vi "GFITS_Str2EXtensions.vi"(8 "error in":errorcluster, 10 "command":string, 11 "curr_ext":i32) -> (0 "error IO":errorcluster, 1 "max_ext":u16=128, 2 "Extensions":i32[](array[numeric]), 3 "geom extensions":i32[](array[numeric]))   [LabVIEW 2016]
panel:
  out "output array":i32[](array[numeric])
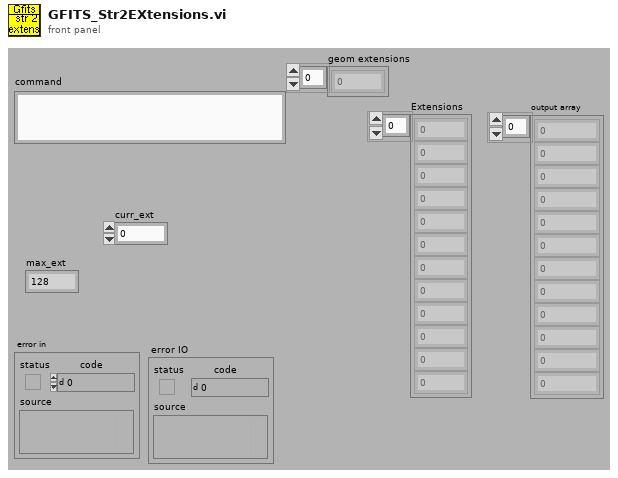
[diagram p1: front panel]
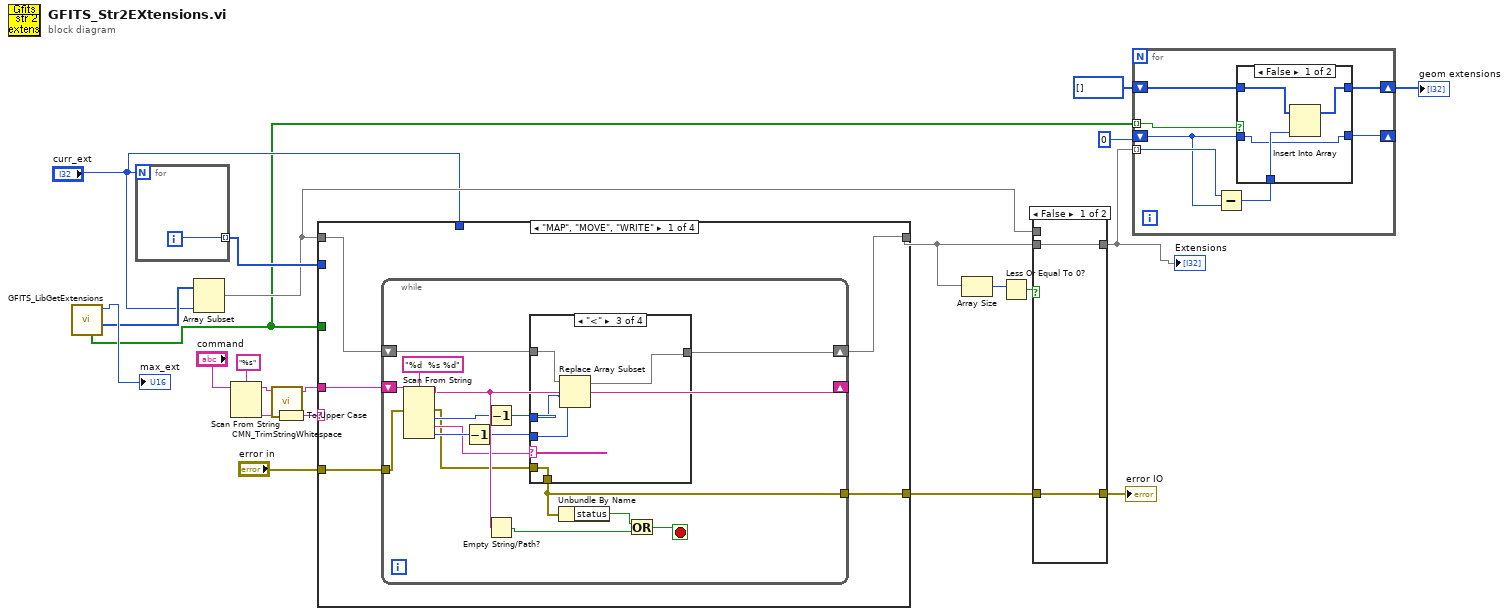
[diagram p0: block diagram]
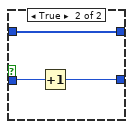
[diagram p2: hidden frame]
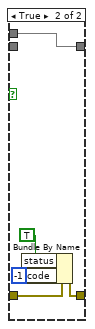
[diagram p3: hidden frame]
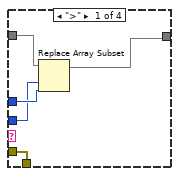
[diagram p4: hidden frame]
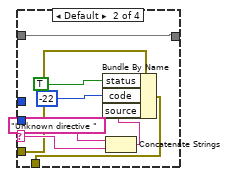
[diagram p5: hidden frame]
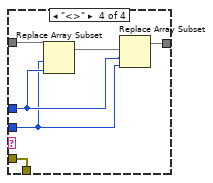
[diagram p6: hidden frame]
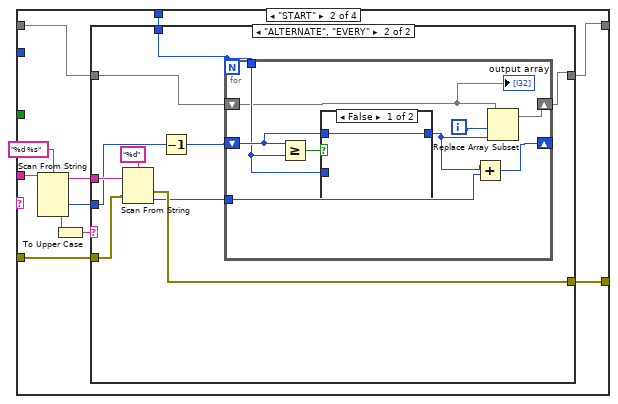
[diagram p7: hidden frame]
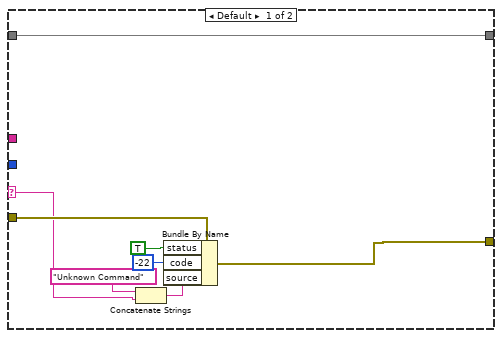
[diagram p8: hidden frame]
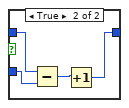
[diagram p9: hidden frame]
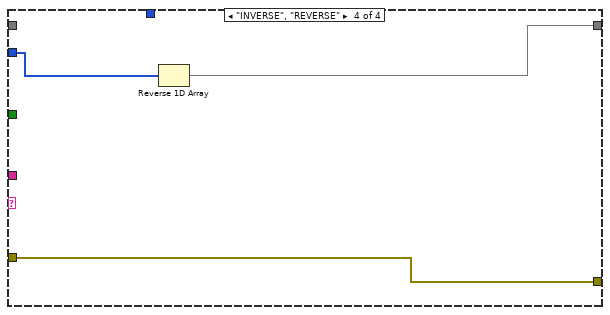
[diagram p11: hidden frame]
diagram:
  n1 = call "GFITS_LibGetExtensions.vi"() -> ("array out"=w8:i32[], "max_ext"=→"max_ext":i32, "discard"=w5:bool[])  [unwired: 2 in, 7 out]
  n2 = for {
    N: "curr_ext" -> [_]
    tunnel: [w23] -> w9 mode=indexing
    i -> [w23]
  }
  n3 = Array Subset(array=w8, length="curr_ext") -> (w7:i32[])  [unwired: 1 in]
  n4 = Scan From String(format string="%s", input string="command") -> (remaining string=w17:string, output 1=w20:string)  [unwired: 2 in, 3 out]
  n5 = call "CMN_TrimStringWhitespace.vi"("string"=w17) -> ("trimmed string"=w16:string)  [unwired: 1 in, 8 out]
  n6 = To Upper Case(1:w20) -> (0:w19:string)
  n7 = case shown="\"MAP\", \"MOVE\", \"WRITE\"" w19 {
    tunnel: w16 -> [w24 w79 _ _]
    tunnel: w7 -> [w28 w71 _ _]
    tunnel: [w27 w70 w112 w114] -> w11
    tunnel: "error in" -> [w26 w73 w113 w116]
    tunnel: [w25 w72 w113 w116] -> w13
    tunnel: "curr_ext" -> [_ w69 _ _]
    tunnel: w9 -> [_ _ w112 w115]
    tunnel: w5 -> [_ _ _ _]
    frame "MAP", "MOVE", "WRITE" {
      n8 = while {
        shift-right: [w42] -> _
        shift-left: w24 -> [w44]
        shift-right: [w40] -> w27
        shift-left: w28 -> [w35]
        tunnel: w26 -> [w31]
        tunnel: [w29] -> w25
        stop <- w32 stop-if-true
        n9 = Scan From String(format string="%d  %s %d", input string=w44, error in=w31) -> (remaining string=w42:string, error out=w30:errorcluster, output 1=w41:i32, output 2=w36:string, output 3=w39:i32)  [unwired: 1 in, 4 out]
        n10 = Decrement(x=w39) -> (x-1=w38:i32)
        n11 = Decrement(x=w41) -> (x-1=w37:i32)
        n12 = Empty String/Path?(string/path=w42) -> (empty?=w34:bool)
        n13 = case shown="\"<\"" w36 {
          selector: w36 -> [_ w53 _ _]
          tunnel: [w48 w57 w61 w68] -> w40
          tunnel: w38 -> [w46 _ w59 w64]
          tunnel: w37 -> [w47 _ w60 w65]
          tunnel: w35 -> [w49 w57 w62 w67]
          tunnel: w30 -> [w45 w51 w58 w63]
          tunnel: [w45 w50 w58 w63] -> w29
          frame ">" {
            n14 = Replace Array Subset(array=w49, new element=w47, index=w46) -> (w48:i32[])
          }
          frame Default {
            n15 = Concatenate Strings("Unknown directive " ("source"), w53) -> (w52:string)
            n16 = Bundle By Name(cluster=w51, "status"=TRUE, "code"=-22, "source"=w52) -> (w50:errorcluster)
          }
          frame "<" {
            n17 = Replace Array Subset(array=w62, new element=w59, index=w60) -> (w61:i32[])
          }
          frame "<>" {
            n18 = Replace Array Subset(array=w67, new element=w65, index=w64) -> (w66:i32[])
            n19 = Replace Array Subset(array=w66, new element=w64, index=w65) -> (w68:i32[])
          }
        }
        n20 = Unbundle By Name(w29) -> ("status"=w33:bool)
        n21 = Or(x=w33, y=w34) -> (x .or. y?=w32:bool)
      }
    }
    frame "START" {
      n22 = Scan From String(format string="%d %s", input string=w79) -> (remaining string=w74:string, output 1=w75:i32, output 2=w77:string)  [unwired: 2 in, 4 out]
      n23 = To Upper Case(1:w77) -> (0:w76:string)
      n24 = case shown="\"ALTERNATE\", \"EVERY\"" w76 {
        selector: w76 -> [w83 _]
        tunnel: w75 -> [_ w90]
        tunnel: w74 -> [_ w97]
        tunnel: w73 -> [w87 w95]
        tunnel: [w81 w94] -> w72
        tunnel: w71 -> [w80 w88]
        tunnel: [w80 w92] -> w70
        tunnel: w69 -> [_ w91]
        frame Default {
          n25 = Concatenate Strings("Unknown Command" ("source"), w83) -> (w82:string)
          n26 = Bundle By Name(cluster=w87, "status"=TRUE, "code"=-22, "source"=w82) -> (w81:errorcluster)
        }
        frame "ALTERNATE", "EVERY" {
          n27 = Scan From String(format string="%d", input string=w97, error in=w95) -> (error out=w94:errorcluster, output 1=w93:i32)  [unwired: 1 in, 3 out]
          n28 = Decrement(x=w90) -> (x-1=w89:i32)
          n29 = for {
            N: w91 -> [_]
            shift-right: [w101] -> w92
            shift-left: w88 -> [w100]
            tunnel: w93 -> [w106]
            tunnel: w91 -> [w102]
            shift-right: [w105] -> _
            shift-left: w89 -> [w104]
            i -> [w99]
            n30 = Greater Or Equal?(x=w104, y=w102) -> (x >= y?=w103:bool)
            n31 = case shown="False" w103 {
              tunnel: w104 -> [w107 w109]
              tunnel: [w107 w110] -> w98
              tunnel: w102 -> [_ w108]
              frame False {
              }
              frame True {
                n32 = Subtract(x=w109, y=w108) -> (x-y=w111:i32)
                n33 = Increment(x=w111) -> (x+1=w110:i32)
              }
            }
            n34 = Add(x=w98, y=w106) -> (x+y=w105:i32)
            n35 = Replace Array Subset(array=w100, new element=w98, index=w99) -> (w101:i32[])
            "output array" <- w100
          }
        }
      }
    }
    frame "ORDERED", Default {
    }
    frame "INVERSE", "REVERSE" {
      n36 = Reverse 1D Array(array=w115) -> (reversed array=w114:i32[])
    }
  }
  n37 = Array Size(array=w11) -> (size(s)=w15:i32)
  n38 = Less Or Equal To 0?(x=w15) -> (x <= 0?=w14:bool)
  n39 = case shown="False" w14 {
    tunnel: w13 -> [w118 w121]
    tunnel: [w118 w120] -> w12
    tunnel: w11 -> [w117 _]
    tunnel: [w117 w119] -> w4
    tunnel: w7 -> [_ w119]
    frame False {
    }
    frame True {
      n40 = Bundle By Name(cluster=w121, "status"=TRUE, "code"=-1) -> (w120:errorcluster)
    }
  }
  "Extensions" <- w4
  "error IO" <- w12
  n41 = for {
    tunnel: w4 -> [w125] mode=indexing
    tunnel: w5 -> [w130] mode=indexing
    shift-right: [w126] -> _
    shift-left: 0 -> [w124]
    shift-right: [w128] -> w2
    shift-left: i32[] [] -> [w127]
    n42 = Subtract(x=w125, y=w124) -> (x-y=w129:i32)
    n43 = case shown="False" w130 {
      tunnel: w129 -> [w134 _]
      tunnel: [w133 w137] -> w128
      tunnel: w127 -> [w132 w137]
      tunnel: w124 -> [w131 w136]
      tunnel: [w131 w135] -> w126
      frame False {
        n44 = Insert Into Array(array=w132, new element=w134) -> (w133:i32[])  [unwired: 1 in]
      }
      frame True {
        n45 = Increment(x=w136) -> (x+1=w135:i32)
      }
    }
  }
  "geom extensions" <- w2
